vi "load_instruments.vi"() -> (3 "output array":string[][](array[string]))   [LabVIEW 2015]
doc: "loads the setup data from the instruments objects"
uses:
  Classes/Instrument/instrument.lvclass
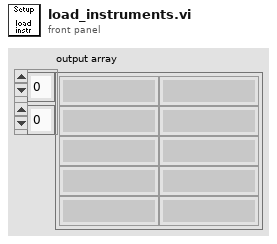
[diagram p1: front panel]
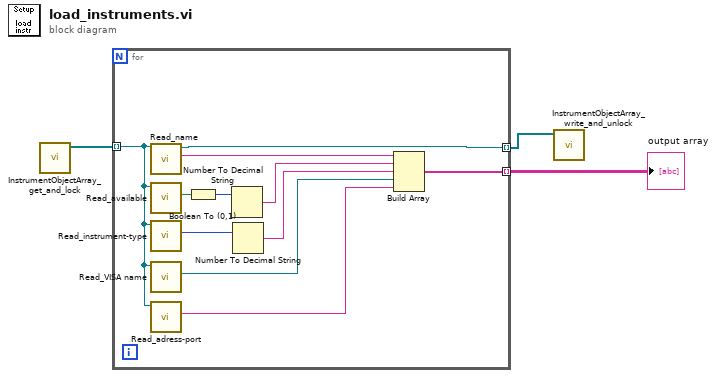
[diagram p0: block diagram]
diagram:
  n1 = call "InstrumentObjectArray_get_and_lock.vi"() -> ("InstrumentsObjects"=w3:refnum<class "instrument.lvclass">[])  [unwired: 10 in, 1 out]
  n2 = for {
    tunnel: w3 -> [w14] mode=indexing
    tunnel: [w5] -> w2 mode=indexing
    tunnel: [w4] -> w1 mode=indexing
    n3 = call-dynamic "Read_name.vi"("instrument in"=w14) -> ("name"=w13:string, "instrument out"=w4:refnum<class "instrument.lvclass">)  [unwired: 8 in, 1 out]
    n4 = call-dynamic "Read_available.vi"("instrument in"=w14) -> ("available?"=w12:bool)  [unwired: 8 in, 2 out]
    n5 = call-dynamic "Read_instrument-type.vi"("instrument in"=w14) -> ("instrument type"=w9:u16)  [unwired: 8 in, 2 out]
    n6 = call-dynamic "Read_VISA name.vi"("instrument in"=w14) -> ("VISA resource name"=w7:refnum<visa-resource-name>)  [unwired: 8 in, 2 out]
    n7 = call "Read_adress-port.vi"("instrument in"=w14) -> ("adress"=w6:string)  [unwired: 7 in, 3 out]
    n8 = Boolean To (0,1)(Boolean=w12) -> (0, 1=w11:i16)
    n9 = Number To Decimal String(number=w11) -> (decimal integer string=w10:string)  [unwired: 1 in]
    n10 = Number To Decimal String(number=w9) -> (decimal integer string=w8:string)  [unwired: 1 in]
    n11 = Build Array(w13, w10, w8, w7, w6) -> (w5:string[])
  }
  "output array" <- w2
  n12 = call "InstrumentObjectArray_write_and_unlock.vi"("InstrumentObjects"=w1) -> ()  [unwired: 10 in, 1 out]
